vi "sub_psk_symbol_map_gen.vi"(9 "Gray code?":bool=TRUE, 11 "M-PSK":i32=4) -> (1 "index map":u32[](array[numeric]), 3 "symbol map":cdb[](array[numeric]))   [LabVIEW 2014]
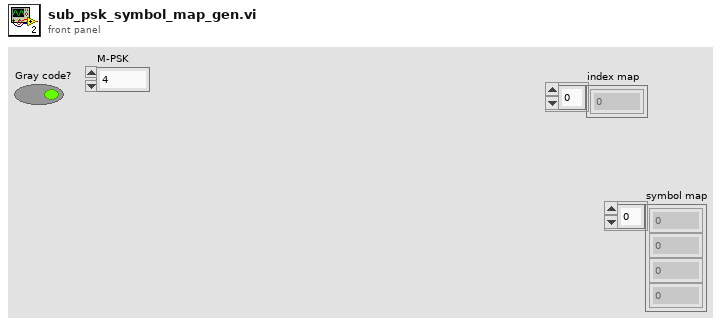
[diagram p1: front panel]
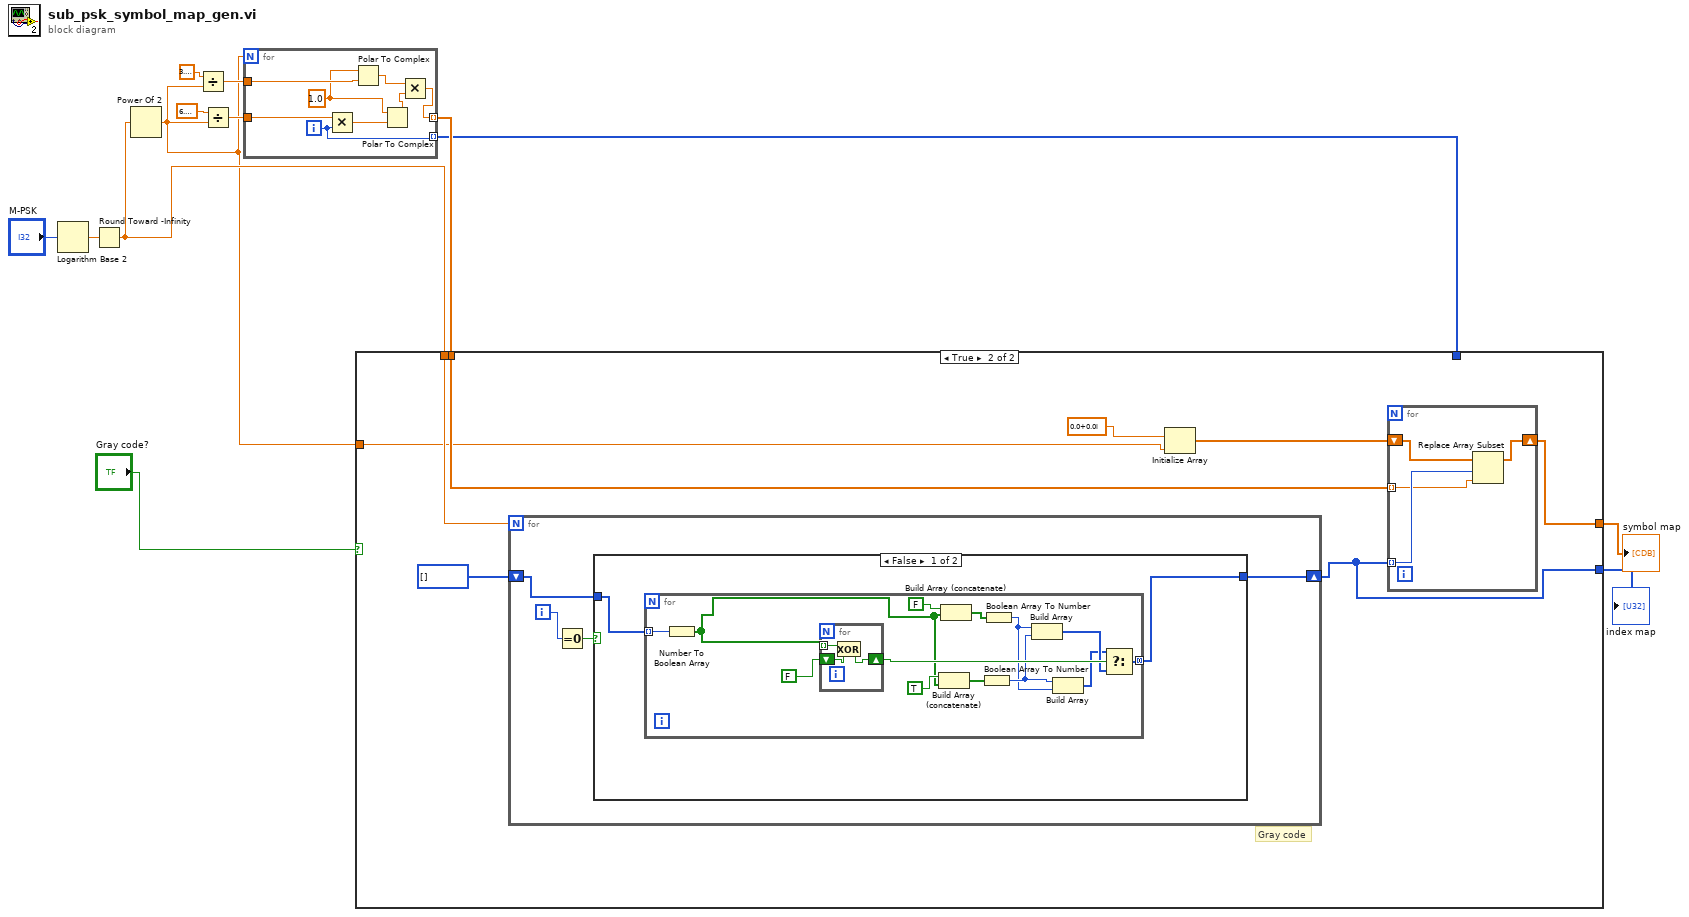
[diagram p0: block diagram]
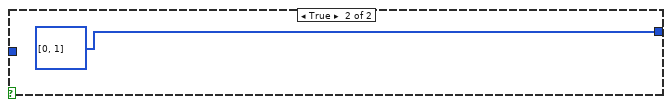
[diagram p3: hidden frame]
diagram:
  n1 = Logarithm Base 2(1:"M-PSK") -> (0:w12:dbl)
  n2 = Round Toward -Infinity(1:w12) -> (0:w9:dbl)
  n3 = Power Of 2(x=w9) -> (2^x=w1:dbl)
  n4 = Divide(x=3.141592653589793, y=w1) -> (x/y=w5:dbl)
  n5 = Divide(x=6.283185307179586, y=w1) -> (x/y=w8:dbl)
  n6 = for {
    N: w1 -> [_]
    tunnel: w8 -> [w21]
    tunnel: [w15] -> w11 mode=indexing
    tunnel: w5 -> [w19]
    tunnel: [w14] -> w3 mode=indexing
    i -> [w14]
    w18 = 1.0 ("r")
    n7 = Multiply(x=w21, y=w14) -> (x*y=w20:dbl)
    n8 = Polar To Complex(1:w19, 2:w18) -> (0:w17:cdb)
    n9 = Polar To Complex(1:w20, 2:w18) -> (0:w16:cdb)
    n10 = Multiply(x=w17, y=w16) -> (x*y=w15:cdb)
  }
  n11 = case shown="True" "Gray code?" {
    tunnel: w11 -> [w23 w26]
    tunnel: [w23 w25] -> w10
    tunnel: w9 -> [_ w28]
    tunnel: [w22 w30] -> w4
    tunnel: w3 -> [w22 _]
    tunnel: w1 -> [_ w24]
    frame False {
    }
    frame True {
      # "Gray code"
      n12 = for {
        N: w28 -> [_]
        shift-right: [w38] -> w30
        shift-left: i32[] [] -> [w37]
        i -> [w36]
        n13 = Equal To 0?(x=w36) -> (x = 0?=w39:bool)
        n14 = case shown="False" w39 {
          tunnel: [w40 i32[] [0, 1]] -> w38
          tunnel: w37 -> [w41 _]
          frame False {
            n15 = for {
              tunnel: w41 -> [w54] mode=indexing
              tunnel: [w45] -> w40 mode=concatenating
              n16 = Number To Boolean Array(number=w54) -> (Boolean array=w44:bool[])
              n17 = for {
                shift-right: [w55] -> w52
                shift-left: FALSE -> [w57]
                tunnel: w44 -> [w56] mode=indexing
                n18 = Exclusive Or(1:w57, 2:w56) -> (0:w55:bool)
              }
              n19 = Build Array (concatenate)(TRUE, w44) -> (w48:bool[])
              n20 = Build Array (concatenate)(FALSE, w44) -> (w49:bool[])
              n21 = Boolean Array To Number(Boolean array=w48) -> (number=w47:u32)
              n22 = Boolean Array To Number(Boolean array=w49) -> (number=w46:u32)
              n23 = Build Array(w46, w47) -> (w43:u32[])
              n24 = Build Array(w47, w46) -> (w42:u32[])
              n25 = Select(t=w42, s=w52, f=w43) -> (s? t:f=w45:u32[])
            }
          }
          frame True {
          }
        }
      }
      n26 = Initialize Array(cdb 0.0+0.0i, w24) -> (w27:cdb[])
      n27 = for {
        tunnel: w30 -> [w34] mode=indexing
        shift-right: [w32] -> w25
        shift-left: w27 -> [w35]
        tunnel: w26 -> [w33] mode=indexing
        n28 = Replace Array Subset(array=w35, new element=w33, index=w34) -> (w32:cdb[])
      }
    }
  }
  "symbol map" <- w10
  "index map" <- w4
